vi "ReportError Event Callback.vi"(4 "TestStand Engine":refnum<k7>, 5 "Event data":cluster{"errorCode":i32, "errorMessage":string}, 6 "CtlRef":refnum<k7>, 7 "Event common data":cluster{"Source":i32, "Type":u32, "Time":u32}) -> ()   [LabVIEW 2025, in "Config Tool.lvlib"]
doc: "The Application Manager generates the ReportError event when TestStand generates an error."
uses:
  Config Tool.lvlib
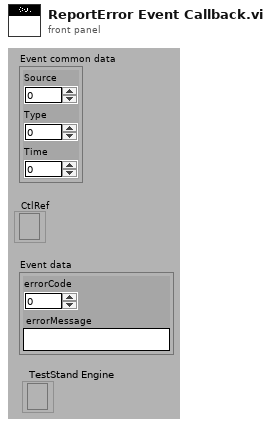
[diagram p1: front panel]
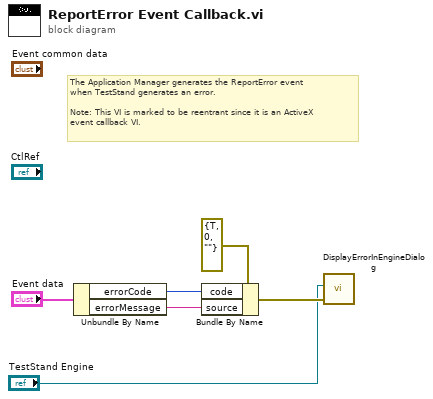
[diagram p0: block diagram]
diagram:
  # "The Application Manager generates the ReportError event\nwhen TestStand generates an error.\n\nNote: This VI is marked to be reentrant since it is an ActiveX\nevent callback VI."
  n1 = Unbundle By Name("Event data") -> ("errorCode"=w4:i32, "errorMessage"=w5:string)
  n2 = Bundle By Name(cluster=errorcluster {"status"=TRUE, "code"=0, "source"=""} ("error in (no error)"), "code"=w4, "source"=w5) -> (w2:errorcluster)
  n3 = call "DisplayErrorInEngineDialog .vi"("error in (no error)"=w2, "TestStand Engine"="TestStand Engine") -> ()  [unwired: 10 in]
